vi "Read Image Size.vi"(8 "error in (no error)":errorcluster, 11 "ImageDistorter in":refnum<class "ImageDistorter.lvclass">) -> (0 "error out":errorcluster, 2 "Image Size":T1, 3 "ImageDistorter out":refnum<class "ImageDistorter.lvclass">)   [LabVIEW 2020, in "image.lvlib" / "ImageDistorter.lvclass"]
uses:
  ImageDistorter.lvclass
  common/Image Size (Integer).ctl
  ImageDistorter.lvclass/ImageDistorter.ctl
  common/common.lvlib
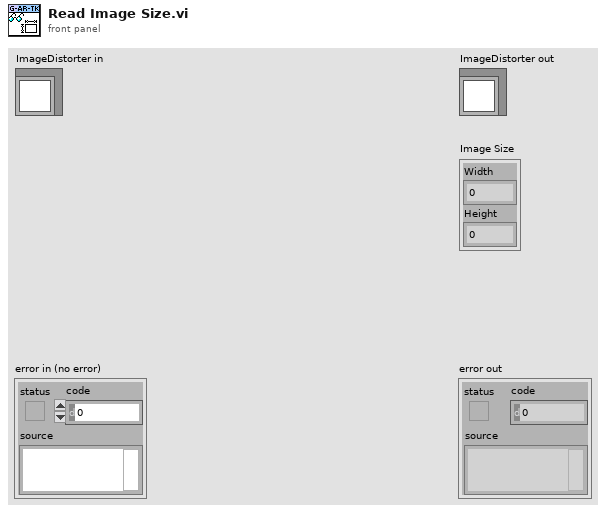
[diagram p1: front panel]
types:
  T1 = typedef "common.lvlib/Image Size (Integer).ctl" = cluster{"Width":u16, "Height":u16}
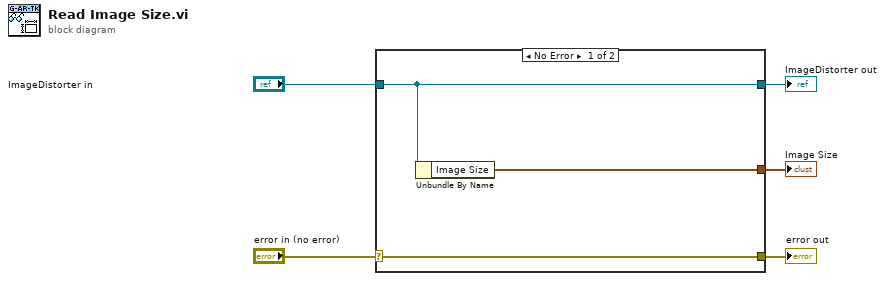
[diagram p0: block diagram]
diagram:
  n1 = case shown="No Error" "error in (no error)" {
    selector: "error in (no error)" -> [w8 w9]
    tunnel: [w8 w9] -> w4
    tunnel: [w7 w10] -> w2
    tunnel: "ImageDistorter in" -> [w7 w10]
    tunnel: [w6 _] -> w1
    frame No Error {
      n2 = Unbundle By Name(w7) -> ("Image Size"=w6:T1)
    }
    frame Error {
    }
  }
  "error out" <- w4
  "ImageDistorter out" <- w2
  "Image Size" <- w1
